vi "DataPacker_Monitor.vi"() -> ()   [LabVIEW 2018, in "feGEM DataPacker.lvlib"]
uses:
  feGEM DataPacker.lvlib
  GlobalVariables/DataPacker_Buffer_Usage_Enum.ctl
  GlobalVariables/Set_And_Get_Enum.ctl
  GlobalVariables/DataPacker_Global_Stop_Enum.ctl
panel:
  in  "Stop Monitor (Keep on logging \nor whever running in background)":bool
  out "Queue Size":i32
  out "# elements in queue":i32
  out "Elements bundled for serialisation":i32
  out "Unique Banks to serialise":i32
  out "?":bool
  out "?":bool
  out "?":bool
  out "Connection Attempt":u32
  out "MIDAS Port out":u16
  out "MIDAS Addresss out":string
  out "Parent VI to the DataPacker Daemon (Main VI name)":string
  out "This Computer Name":string
  out "Hard Stop?\n(Stop Executing)":bool
  out "Soft Stop?\n(Stop Requested)":bool
  out "Average MIDAS Processing Time (ms)":dbl(knob) scale=1.0..1000.0
  out "Last Midas Handling Time (ms)":dbl(knob) scale=0.0..10.0
  out "Seconds since last \ncommunication with\\\nMIDAS":dbl
  out "MIDAS Connection OK":bool
  out "DataPacker Queue Usage (%)":dbl(knob) scale=0.0..100.0
  out "MIDAS Buffer Usage (%)":dbl(knob) scale=0.0..100.0
  out "Time since last sleep (ms)":dbl(knob) scale=1.0..1000.0
  out "Time Bundling Data (Reading from Queue into LV structures)":dbl(knob) scale=0.0..100.0
  out "% Time Packing (Serializing Queued Data)":dbl(knob) scale=0.0..100.0
  in  "Debug Mode":bool
  out "MIDAS Reply (Requires debug mode to be on)":string
  # "MIDAS side processing speeds"
  # "Bandwidth usage / Memory usage"
  # "Local processing speeds"
  # "Global stop variables (FGV)"
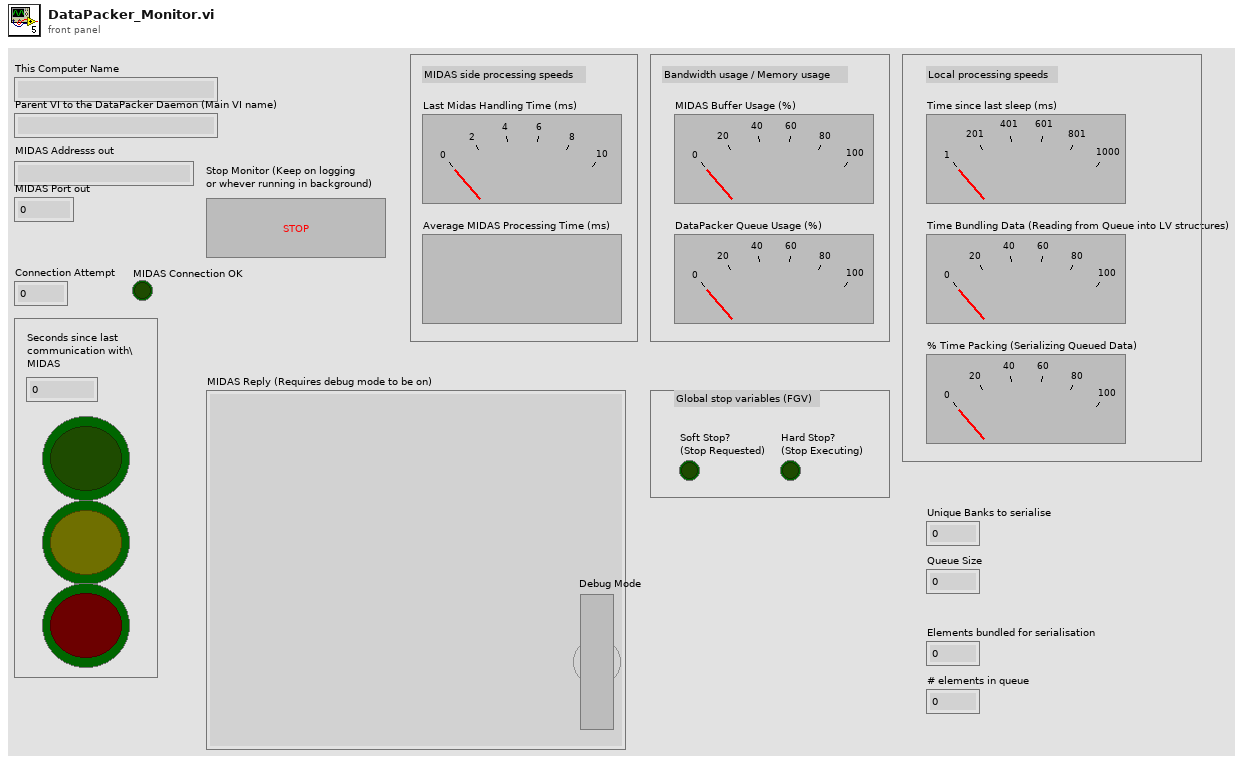
[diagram p1: front panel]
types:
  T1 = typedef "feGEM DataPacker.lvlib/Set_And_Get_Enum.ctl" = enum16{"Set", "Get"}
  T2 = typedef "feGEM DataPacker.lvlib/DataPacker_Global_Stop_Enum.ctl" = enum16{"Reset", "Set Soft Stop", "Get Soft Stop", "Set Hard Stop", "Get Hard Stop", "Get Any Stop"}
  T3 = typedef "feGEM DataPacker.lvlib/DataPacker_Buffer_Usage_Enum.ctl" = enum16{"Get Values", "Set MIDAS Buffer Usage (%)", "Set DataPacker Queue\nUsage (%)"}
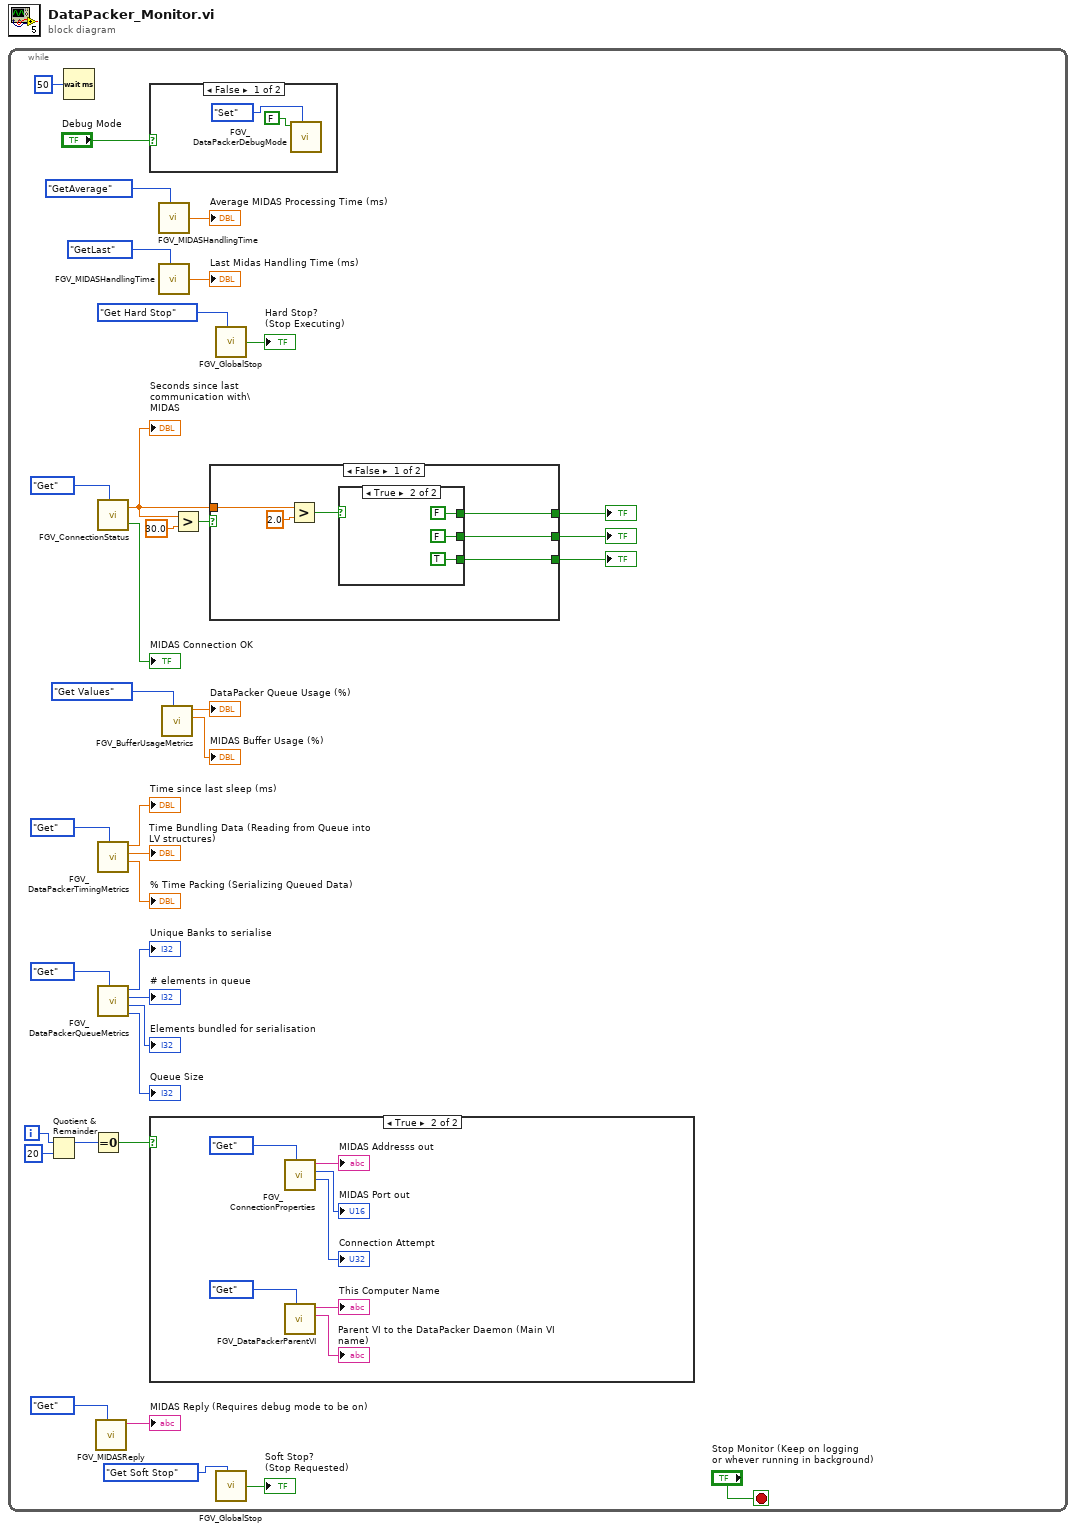
[diagram p0: block diagram]
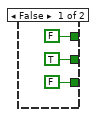
[diagram p3: hidden frame]
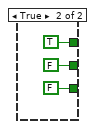
[diagram p4: hidden frame]
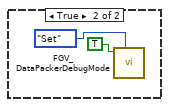
[diagram p5: hidden frame]
diagram:
  n1 = while {
    i -> [w4]
    stop <- "Stop Monitor (Keep on logging \nor whever running in background)" stop-if-true
    n2 = Quotient & Remainder(x=w4, y=20) -> (x-y*floor(x/y)=w2:i32)  [unwired: 1 out]
    n3 = Wait (ms)(milliseconds to wait=u32 50) -> ()  [unwired: 1 out]
    n4 = Equal To 0?(x=w2) -> (x = 0?=w1:bool)
    n5 = call "FGV_MIDASReply.vi"("Enum"=Set_And_Get_Enum."Get") -> ("MIDAS Reply"=→"MIDAS Reply (Requires debug mode to be on)":string)  [unwired: 10 in]
    n6 = call "FGV_ConnectionStatus.vi"("Enum"=enum16{"Get", "Set"}."Get") -> ("Seconds since last communication with MIDAS"=w11:dbl, "MIDAS Connection OK"=→"MIDAS Connection OK":bool)  [unwired: 4 in]
    "Seconds since last \ncommunication with\\\nMIDAS" <- w11
    n7 = call "FGV_DataPackerTimingMetrics.vi"(7:Set_And_Get_Enum."Get") -> ("% Time Packing (Serializing Queued Data)"=→"% Time Packing (Serializing Queued Data)":dbl, "Time Bundling Data (Reading from Queue into LV structures)"=→"Time Bundling Data (Reading from Queue into LV structures)":dbl, "Time since last sleep (ms)"=→"Time since last sleep (ms)":dbl)  [unwired: 8 in]
    n8 = call "FGV_DataPackerQueueMetrics.vi"("Enum"=Set_And_Get_Enum."Get") -> ("Queue Size"=→"Queue Size":i32, "Elements bundled for serialisation"=→"Elements bundled for serialisation":i32, "# elements in queue"=→"# elements in queue":i32, "Unique Banks to serialise"=→"Unique Banks to serialise":i32)  [unwired: 7 in]
    n9 = case shown="False" "Debug Mode" {
      frame False {
        n10 = call "FGV_DataPackerDebugMode.vi"(7:Set_And_Get_Enum."Set", "Boolean"=FALSE) -> ()  [unwired: 9 in, 1 out]
      }
      frame True {
        n11 = call "FGV_DataPackerDebugMode.vi"(7:Set_And_Get_Enum."Set", "Boolean"=TRUE) -> ()  [unwired: 9 in, 1 out]
      }
    }
    n12 = case shown="True" w1 {
      frame False {
      }
      frame True {
        n13 = call "FGV_ConnectionProperties.vi"("Enum"=Set_And_Get_Enum."Get") -> ("Connection Attempt out"=→"Connection Attempt":u32, "MIDAS Port out"=→"MIDAS Port out":u16, "MIDAS Addresss out"=→"MIDAS Addresss out":string)  [unwired: 7 in, 1 out]
        n14 = call "FGV_DataPackerParentVI.vi"("Enum"=Set_And_Get_Enum."Get") -> ("Parent VI to the DataPacker Daemon (Main VI name)"=→"Parent VI to the DataPacker Daemon (Main VI name)":string, "This Computer Name"=→"This Computer Name":string)  [unwired: 9 in]
      }
    }
    n15 = call "FGV_MIDASHandlingTime.vi"("Enum"=enum16{"Set", "GetLast", "GetAverage"}."GetAverage") -> ("Midas Handling Time"=→"Average MIDAS Processing Time (ms)":dbl)  [unwired: 4 in]
    n16 = call "FGV_MIDASHandlingTime.vi"("Enum"=enum16{"Set", "GetLast", "GetAverage"}."GetLast") -> ("Midas Handling Time"=→"Last Midas Handling Time (ms)":dbl)  [unwired: 4 in]
    n17 = call "FGV_BufferUsageMetrics.vi"(7:DataPacker_Buffer_Usage_Enum."Get Values") -> ("MIDAS Buffer Usage (%)"=→"MIDAS Buffer Usage (%)":dbl, "DataPacker Queue Usage (%)"=→"DataPacker Queue Usage (%)":dbl)  [unwired: 9 in]
    n18 = Greater?(x=w11, y=30.0) -> (0:w12:bool)
    n19 = case shown="False" w12 {
      tunnel: [w46 FALSE] -> w15
      tunnel: [w48 FALSE] -> w14
      tunnel: [w47 TRUE] -> w13
      tunnel: w11 -> [w50 _]
      frame False {
        n20 = Greater?(x=w50, y=2.0) -> (0:w45:bool)
        n21 = case shown="True" w45 {
          tunnel: [TRUE FALSE] -> w48
          tunnel: [FALSE FALSE] -> w47
          tunnel: [FALSE TRUE] -> w46
          frame False {
          }
          frame True {
          }
        }
      }
      frame True {
      }
    }
    "?" <- w14
    "?" <- w15
    "?" <- w13
    n22 = call "FGV_GlobalStop.vi"("Enum"=DataPacker_Global_Stop_Enum."Get Hard Stop") -> ("Stop"=→"Hard Stop?\n(Stop Executing)":bool)  [unwired: 4 in]
    n23 = call "FGV_GlobalStop.vi"("Enum"=DataPacker_Global_Stop_Enum."Get Soft Stop") -> ("Stop"=→"Soft Stop?\n(Stop Requested)":bool)  [unwired: 4 in]
  }
